vi "Set All Gear Ratio.vi"(8 "error in (no error)":errorcluster, 9 "gear ratio":dbl[](array[numeric]), 10 "wheel indexes":i32[](array[numeric]), 11 "steering frame in":refnum<class "NI_Robotics_Steering Frame.lvclass">) -> (0 "error out":errorcluster, 1 "found?":bool[](array[boolean]), 3 "steering frame out":refnum<class "NI_Robotics_Steering Frame.lvclass">)   [LabVIEW 2017, in "NI_Robotics_Steering Frame.lvclass"]
uses:
  <vilib>/robotics/Steering/Steering Frame/NI_Robotics_Steering Frame.lvclass
  <vilib>/robotics/Steering/Steering Frame/NI_Robotics_Steering Frame.lvclass/NI_Robotics_Steering Frame.ctl
  <vilib>/robotics/Steering/Wheel/NI_Robotics_Wheel.lvclass/NI_Robotics_Wheel.ctl
  <vilib>/robotics/Steering/Wheel/Update Steering to Wheel Frame Transform.vi
  <vilib>/Analysis/coordinate.llb/Wrap Angle.vi
  <vilib>/Analysis/coordinate.llb/Wrap Angle (scalar).vi
  <vilib>/robotics/Steering/Wheel/Get Wheel Name.vi
  <vilib>/robotics/Steering/Wheel/NI_Robotics_Wheel.lvclass
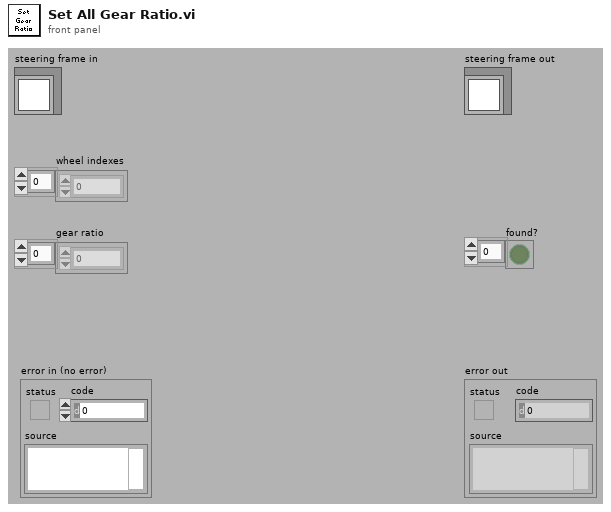
[diagram p1: front panel]
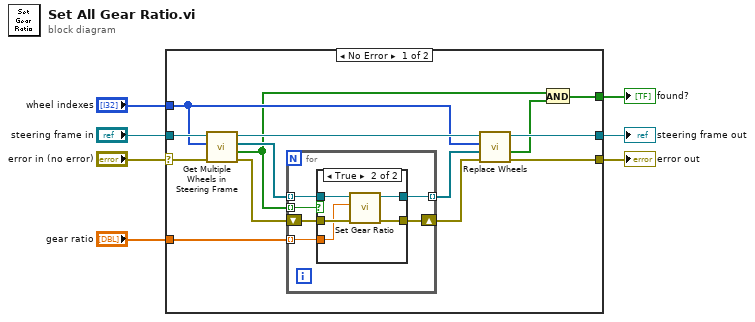
[diagram p0: block diagram]
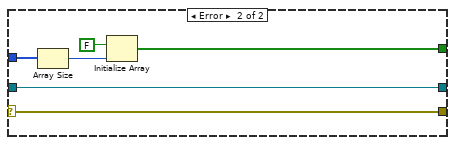
[diagram p3: hidden frame]
diagram:
  n1 = case shown="No Error" "error in (no error)" {
    selector: "error in (no error)" -> [w20 w40]
    tunnel: [w11 w40] -> w6
    tunnel: [w12 w39] -> w4
    tunnel: "steering frame in" -> [w21 w39]
    tunnel: "wheel indexes" -> [w15 w36]
    tunnel: "gear ratio" -> [w16 _]
    tunnel: [w8 w35] -> w1
    frame No Error {
      n2 = call <vilib>:"Get Multiple Wheels in Steering Frame.vi"("error in (no error)"=w20, "wheel indexes"=w15, "steering frame in"=w21) -> ("error out"=w17:errorcluster, "found?"=w10:bool[], "wheels"=w19:refnum<class "NI_Robotics_Wheel.lvclass">[], "steering frame out"=w18:refnum<class "NI_Robotics_Steering Frame.lvclass">)  [unwired: 2 in, 3 out]
      n3 = for {
        tunnel: w19 -> [w27] mode=indexing
        tunnel: w16 -> [w25] mode=indexing
        tunnel: [w24] -> w14 mode=indexing
        shift-right: [w23] -> w13
        shift-left: w17 -> [w26]
        tunnel: w10 -> [w22] mode=indexing
        n4 = case shown="True" w22 {
          tunnel: w27 -> [w29 w34]
          tunnel: w26 -> [w28 w33]
          tunnel: w25 -> [_ w32]
          tunnel: [w29 w31] -> w24
          tunnel: [w28 w30] -> w23
          frame False {
          }
          frame True {
            n5 = call <vilib>:"Set Gear Ratio.vi"("error in (no error)"=w33, "gear ratio"=w32, "wheel in"=w34) -> ("error out"=w30:errorcluster, "wheel out"=w31:refnum<class "NI_Robotics_Wheel.lvclass">)  [unwired: 7 in]
          }
        }
      }
      n6 = call <vilib>:"Replace Wheels.vi"("error in (no error)"=w13, "wheels"=w14, "wheel indexes"=w15, "steering frame in"=w18) -> ("error out"=w11:errorcluster, "found?"=w9:bool[], "steering frame out"=w12:refnum<class "NI_Robotics_Steering Frame.lvclass">)  [unwired: 5 in]
      n7 = And(x=w10, y=w9) -> (x .and. y?=w8:bool[])
    }
    frame Error {
      n8 = Array Size(array=w36) -> (size(s)=w38:i32)
      n9 = Initialize Array(FALSE, w38) -> (w35:bool[])
    }
  }
  "error out" <- w6
  "steering frame out" <- w4
  "found?" <- w1
